vi "Configure Modulation (PM).vi"(0 "VISA resource name":refnum<visa-resource-name>, 1 "Enable PM (T: Enable)":bool=TRUE, 2 "Modulation Waveform (0: Sine)":u16(ring) items=["Sine", "Square", "Ramp", "Noise", "User Waveform", "Edit Memory", "EFile"], 3 "Peak Deviation Unit (0: Radian)":u16(ring) items=["Radians", "Degrees"], 5 "Channel (1: Channel 1)":u16(ring)=1 items=["Channel 1"=1, "Channel 2"=2], 7 "PM Source (0: Internal)":u16(ring) items=["Internal", "External"], 9 "Peak Deviation (0)":dbl, 11 "error in (no error)":errorcluster, 12 "Modulation Frequency (100.00 Hz)":dbl=100.0, 13 "User Waveform (0)":i32, 14 "EFile Name (\"\")":string) -> (4 "VISA resource name out":refnum<visa-resource-name>, 15 "error out":errorcluster)   [LabVIEW 2016, in "Tektronix AFG 1000 Series.lvlib"]
doc: "Configures and enables phase modulation (PM)."
uses:
  Tektronix AFG 1000 Series.lvlib
panel:
  # "Internal PM Settings"
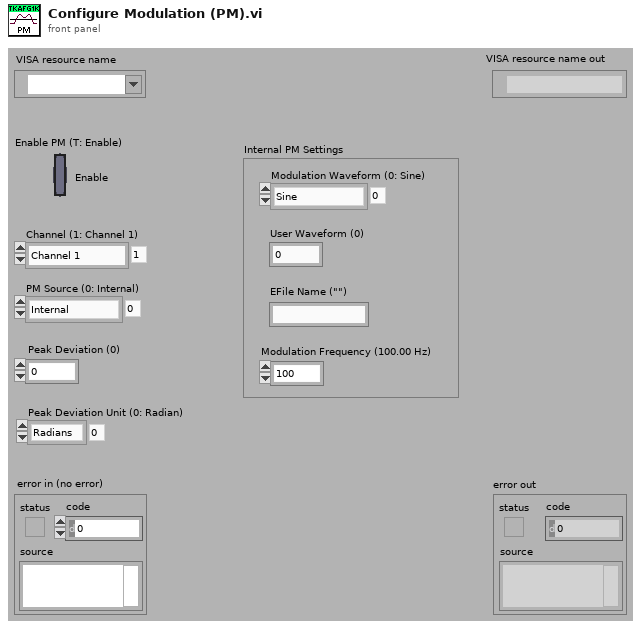
[diagram p1: front panel]
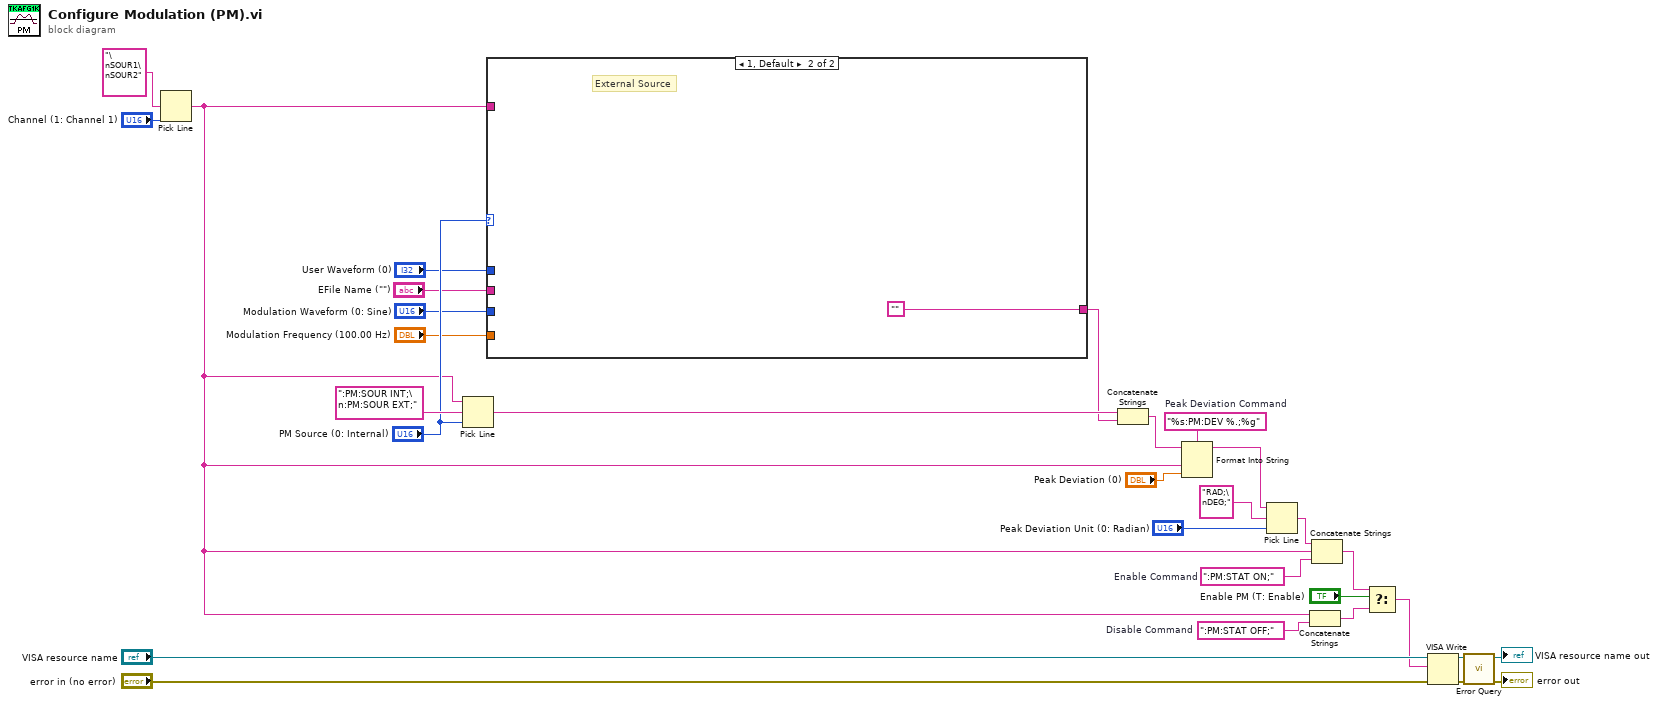
[diagram p0: block diagram]
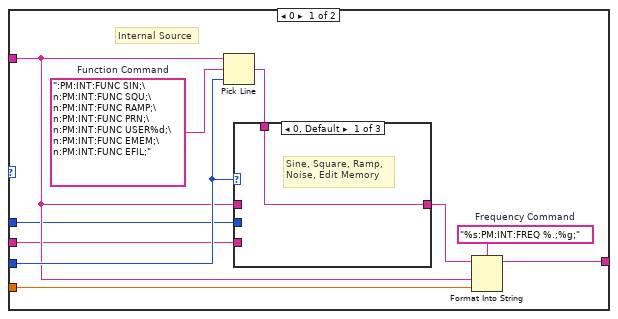
[diagram p2: hidden frame]
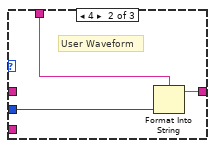
[diagram p3: hidden frame]
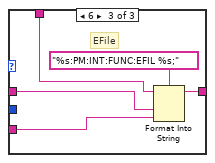
[diagram p4: hidden frame]
diagram:
  w22 = ":PM:STAT ON;"  # Enable Command
  w24 = "%s:PM:DEV %.;%g"  # Peak Deviation Command
  w19 = ":PM:STAT OFF;"  # Disable Command
  n1 = Pick Line(multi-line string="\nSOUR1\nSOUR2" ("string (\"\")"), line index="Channel (1: Channel 1)") -> (output string=w6:string)  [unwired: 1 in]
  n2 = Pick Line(string ("")=w6, multi-line string=":PM:SOUR INT;\n:PM:SOUR EXT;" ("Source Command"), line index="PM Source (0: Internal)") -> (output string=w13:string)
  n3 = case shown="1, Default" "PM Source (0: Internal)" {
    tunnel: w6 -> [w33 _]
    tunnel: [w38 ""] -> w7
    tunnel: "Modulation Waveform (0: Sine)" -> [w34 _]
    tunnel: "Modulation Frequency (100.00 Hz)" -> [w37 _]
    tunnel: "User Waveform (0)" -> [w32 _]
    tunnel: "EFile Name (\"\")" -> [w31 _]
    frame 0 {
      w39 = "%s:PM:INT:FREQ %.;%g;"  # Frequency Command
      w40 = ":PM:INT:FUNC SIN;\n:PM:INT:FUNC SQU;\n:PM:INT:FUNC RAMP;\n:PM:INT:FUNC PRN;\n:PM:INT:FUNC USER%d;\n:PM:INT:FUNC EMEM;\n:PM:INT:FUNC EFIL;"  # Function Command
      # "Internal Source"
      n4 = Pick Line(string ("")=w33, multi-line string=w40, line index=w34) -> (output string=w36:string)
      n5 = case shown="0, Default" w34 {
        tunnel: w36 -> [w41 w44 w48]
        tunnel: [w41 w43 w49] -> w35
        tunnel: w33 -> [_ _ w46]
        tunnel: w32 -> [_ w42 _]
        tunnel: w31 -> [_ _ w45]
        frame 0, Default {
          # "Sine, Square, Ramp,\nNoise, Edit Memory"
        }
        frame 4 {
          # "User Waveform"
          n6 = Format Into String(format string=w44, w42) -> (resulting string=w43:string)  [unwired: 2 in, 1 out]
        }
        frame 6 {
          # "EFile"
          n7 = Format Into String(format string="%s:PM:INT:FUNC:EFIL %s;", initial string=w48, w46, w45) -> (resulting string=w49:string)  [unwired: 1 in, 1 out]
        }
      }
      n8 = Format Into String(format string=w39, initial string=w35, w33, w37) -> (resulting string=w38:string)  [unwired: 1 in, 1 out]
    }
    frame 1, Default {
      # "External Source"
    }
  }
  n9 = Concatenate Strings(w13, w7) -> (w12:string)
  n10 = Format Into String(format string=w24, initial string=w12, w6, "Peak Deviation (0)") -> (resulting string=w2:string)  [unwired: 1 in, 1 out]
  n11 = Pick Line(string ("")=w2, multi-line string="RAD;\nDEG;", line index="Peak Deviation Unit (0: Radian)") -> (output string=w1:string)
  n12 = Concatenate Strings(w6, w19) -> (w17:string)
  n13 = Concatenate Strings(w1, w6, w22) -> (w15:string)
  n14 = Select(t=w15, s="Enable PM (T: Enable)", f=w17) -> (s? t:f=w16:string)
  n15 = VISA Write(VISA resource name="VISA resource name", write buffer=w16, error in (no error)="error in (no error)") -> (VISA resource name out=w27:refnum<visa-resource-name>, error out=w28:errorcluster)  [unwired: 1 out]
  n16 = call "Error Query.vi"("error in (no error)"=w28, "VISA resource name"=w27) -> ("error out"=→"error out":errorcluster, "VISA resource name out"=→"VISA resource name out":refnum<visa-resource-name>)  [unwired: 6 in, 2 out]
